vi "TW Fix VI Missing Paths.vi"(7 "vi reference":refnum<vi>, 8 "error in (no error)":errorcluster, 9 "Replace Subname":string, 10 "New Subname":string, 11 "VI Path":path) -> (0 "error out":errorcluster)   [LabVIEW 2021, in "LV Scripting Utilities.lvlib"]
uses:
  LV Scripting Utilities.lvlib
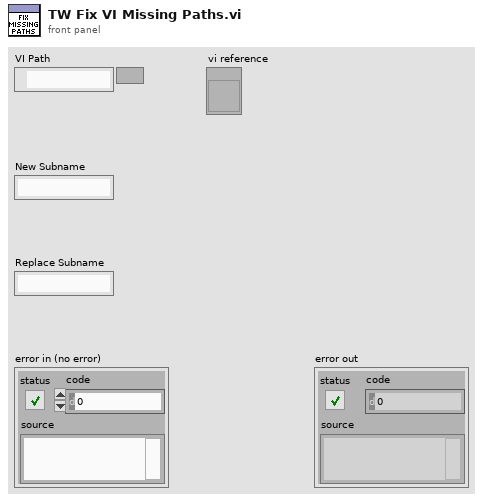
[diagram p1: front panel]
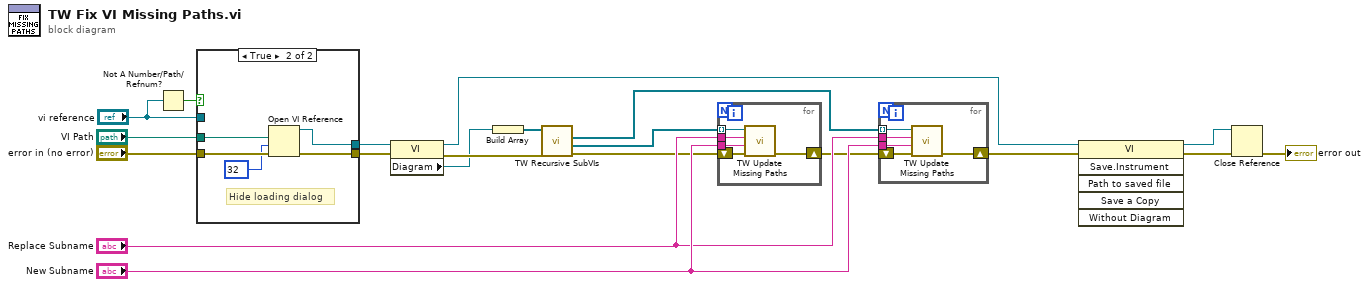
[diagram p0: block diagram]
diagram:
  n1 = Not A Number/Path/Refnum?(number/path/refnum="vi reference") -> (NaN/Path/Refnum?=w1:bool)
  n2 = case shown="True" w1 {
    tunnel: "error in (no error)" -> [w21 w27]
    tunnel: [w21 w26] -> w9
    tunnel: [w22 w25] -> w8
    tunnel: "VI Path" -> [_ w24]
    tunnel: "vi reference" -> [w22 _]
    frame False {
    }
    frame True {
      # "Hide loading dialog"
      n3 = Open VI Reference(vi path=w24, options=32, error in (no error)=w27) -> (vi reference=w25:refnum<vi>, error out=w26:errorcluster)  [unwired: 3 in]
    }
  }
  n4 = property class="VI"(reference=w8, error in=w9) -> (reference out=w5:refnum<vi>, error out=w14:errorcluster, "Diagram"=w12:refnum<vi>)
  n5 = Build Array(w12) -> (w13:refnum<vi>[])
  n6 = call "TW Recursive SubVIs.vi"("error in (no error)"=w14, "Diagrams in"=w13) -> ("error out"=w16:errorcluster, "Constant references out"=w15:refnum<vi>[], "SubVI references out"=w18:refnum<vi>[])  [unwired: 7 in]
  n7 = for {
    tunnel: w15 -> [w32] mode=indexing
    shift-right: [w30] -> w17
    shift-left: w16 -> [w31]
    tunnel: "Replace Subname" -> [w29]
    tunnel: "New Subname" -> [w28]
    n8 = call "TW Update Missing Paths.vi"("error in (no error)"=w31, "New Subname"=w28, "Subname to Replace"=w29, "GObject in"=w32) -> ("error out"=w30:errorcluster)  [unwired: 7 in]
  }
  n9 = for {
    tunnel: w18 -> [w37] mode=indexing
    shift-right: [w35] -> w6
    shift-left: w17 -> [w36]
    tunnel: "Replace Subname" -> [w34]
    tunnel: "New Subname" -> [w33]
    n10 = call "TW Update Missing Paths.vi"("error in (no error)"=w36, "New Subname"=w33, "Subname to Replace"=w34, "GObject in"=w37) -> ("error out"=w35:errorcluster)  [unwired: 7 in]
  }
  n11 = invoke class="VI" method="Save.Instrument"(reference=w5, error in=w6) -> (reference out=w3:refnum<vi>, error out=w4:errorcluster)  [unwired: 4 in, 4 out]
  n12 = Close Reference(reference=w3, error in (no error)=w4) -> (error out=→"error out":errorcluster)
